vi "PicoScope2000RunBlock.vi"(5 "Buffer and Transfer Settings":T1={"startIndex"=0, "Samples"=3968, "Down Sample Ratio"=1, "Down-Sample Mode"=4} {"Down-Sample Mode" items=["RAW none"=2147483648, "None"=0, "Aggregate"=1, "Decimate"=2, "Average"=4]; "Down Sample Ratio" step=1; "Samples" format="%_6p"}, 7 "Acquisition Settings":T2={"preTriggerSamples"=0, "postTriggerSamples"=3968, "timebase"=5} {"postTriggerSamples" format="%_6p"; "preTriggerSamples" format="%_6p"}, 8 "error in (no error)":errorcluster, 11 "handle in":i16=1) -> (0 "error out":errorcluster, 3 "handle out":i16=1, 4 "timeIndisposedMs":dbl=2.0, 6 "Total Requested Samples":u64=1000)   [LabVIEW 2010]
doc: "Calls ps5000aRunBlock"
uses:
  ps2000.dll
  shared/Acquisition Settings.ctl
  shared/Buffer and Transfer Settings.ctl
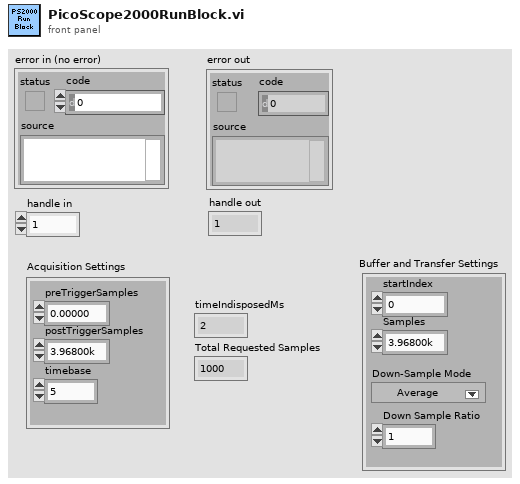
[diagram p1: front panel]
types:
  T1 = typedef "Buffer and Transfer Settings.ctl" = cluster{"startIndex":u64, "Samples":u64, "Down Sample Ratio":u64, "Down-Sample Mode":u32}
  T2 = typedef "Acquisition Settings.ctl" = cluster{"preTriggerSamples":u64, "postTriggerSamples":u64, "timebase":u32}
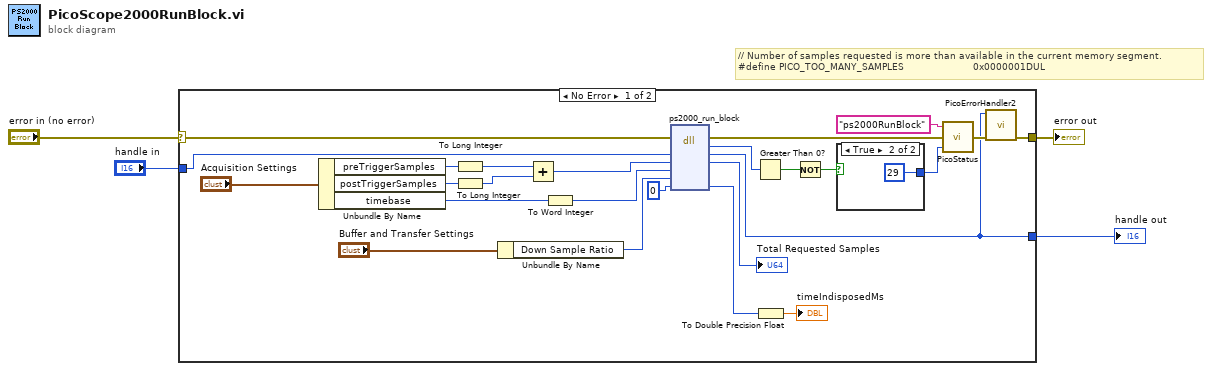
[diagram p0: block diagram]
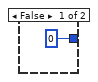
[diagram p2: hidden frame]
diagram:
  # "// Number of samples requested is more than available in the current memory segment.\n#define PICO_TOO_MANY_SAMPLES                       0x0000001DUL"
  n1 = case shown="No Error" "error in (no error)" {
    selector: "error in (no error)" -> [w26 w33]
    tunnel: [w23 w33] -> w2
    tunnel: "handle in" -> [w25 w32]
    tunnel: [w14 w32] -> w3
    frame No Error {
      n2 = Unbundle By Name("Acquisition Settings") -> ("preTriggerSamples"=w22:u64, "postTriggerSamples"=w20:u64, "timebase"=w21:u32)
      n3 = To Long Integer(number=w22) -> (32bit integer=w18:i32)
      n4 = To Long Integer(number=w20) -> (32bit integer=w19:i32)
      n5 = Unbundle By Name("Buffer and Transfer Settings") -> ("Down Sample Ratio"=w9:u64)
      n6 = Add(x=w18, y=w19) -> (x+y=w17:i32)
      n7 = To Word Integer(number=w21) -> (16bit integer=w16:i16)
      n8 = dll-call lib="PS2000.dll" fn="ps2000_run_block"(error in=w26, "handle"=w25, "no_of_samples"=w17, "timebase"=w16, "oversample"=w9, "time_indisposed_ms"=0) -> (error out=w28:errorcluster, "return type"=w12:i16, "handle"=w14:i16, "no_of_samples"=→"Total Requested Samples":i32, "time_indisposed_ms"=w10:i32)  [unwired: 4 in, 1 out]
      n9 = Greater Than 0?(x=w12) -> (x > 0?=w7:bool)
      n10 = To Double Precision Float(number=w10) -> (double precision float=→"timeIndisposedMs":dbl)
      n11 = Not(x=w7) -> (.not. x?=w6:bool)
      n12 = case shown="True" w6 {
        tunnel: [u32 0 ("PICO STATUS") u32 29 ("PICO STATUS")] -> w5
        frame False {
        }
        frame True {
        }
      }
      n13 = call "PicoStatus.vi"("PICO STATUS"=w5, "error in"=w28, "source"="ps2000RunBlock") -> ("error out"=w24:errorcluster)
      n14 = call "PicoErrorHandler2.vi"("error in (no error)"=w24, "handle In"=w14) -> ("error out"=w23:errorcluster)  [unwired: 9 in]
    }
    frame Error {
    }
  }
  "error out" <- w2
  "handle out" <- w3
